vi "Query Motor Speed.vi"(7 "Mono System # (0)":T1, 8 "error in (no error)":errorcluster, 11 "VISA resource name":refnum<visa-resource-name>) -> (0 "error out":errorcluster, 1 "Max Frequency":dbl[unit], 2 "Min Frequency":dbl[unit], 3 "VISA resource name out":refnum<visa-resource-name>, 4 "Ramp Time":dbl[unit])   [LabVIEW 2009, in "JY-SPEX-TRIAX.lvlib"]
doc: "Queries the minimum and maximum motor speeds and the time to ramp from the min to the max."
uses:
  JY-SPEX-TRIAX.lvlib
  controls.llb/Monochromator System Number.ctl
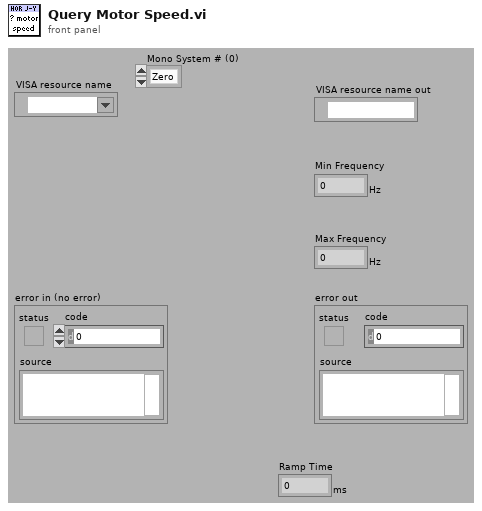
[diagram p1: front panel]
types:
  T1 = typedef "JY-SPEX-TRIAX.lvlib/Monochromator System Number.ctl" = enum16{"Zero", "One"}
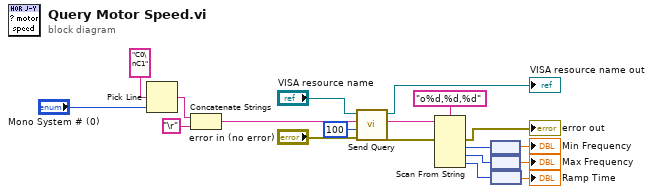
[diagram p0: block diagram]
diagram:
  n1 = Pick Line(multi-line string="C0\nC1", line index="Mono System # (0)") -> (output string=w15:string)  [unwired: 1 out]
  n2 = Concatenate Strings(w15, "\r") -> (w13:string)
  n3 = call "Send Query.vi"("error in (no error)"="error in (no error)", "byte count"=u32 100, "write buffer"=w13, "VISA resource name"="VISA resource name") -> ("error out"=w3:errorcluster, "read buffer"=w11:string, "VISA resource name out"=→"VISA resource name out":refnum<visa-resource-name>)  [unwired: 5 out]
  n4 = Scan From String(format string="o%d,%d,%d", input string=w11, error in=w3) -> (error out=→"error out":errorcluster, output 1=w9:i32, output 2=w8:i32, output 3=w7:i32)  [unwired: 1 in, 5 out]
  n5 = node(w9) -> (→"Min Frequency":dbl[unit])
  n6 = node(w8) -> (→"Max Frequency":dbl[unit])
  n7 = node(w7) -> (→"Ramp Time":dbl[unit])
